vi "_AllThings.vi"   [LabVIEW 2017]
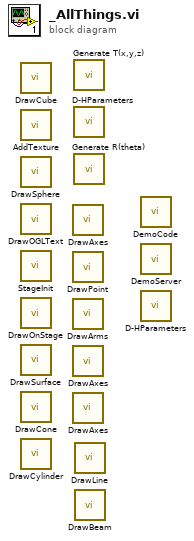
[diagram p0: block diagram]
diagram:
  n1 = call <userlib>:"DrawCube.vi"() -> ()  [unwired: 6 in, 2 out]
  n2 = call <userlib>:"AddTexture.vi"() -> ()  [unwired: 4 in, 2 out]
  n3 = call <userlib>:"DrawSphere.vi"() -> ()  [unwired: 6 in, 2 out]
  n4 = call <userlib>:"DrawOGLText.vi"() -> ()  [unwired: 6 in, 2 out]
  n5 = call <userlib>:"StageInit.vi"() -> ()  [unwired: 4 in, 2 out]
  n6 = call <userlib>:"DrawOnStage.vi"() -> ()  [unwired: 3 in, 3 out]
  n7 = call <userlib>:"DrawSurface.vi"() -> ()  [unwired: 6 in, 2 out]
  n8 = call <userlib>:"DrawCone.vi"() -> ()  [unwired: 6 in, 2 out]
  n9 = call <userlib>:"DrawCylinder.vi"() -> ()  [unwired: 6 in, 2 out]
  n10 = call <userlib>:"DrawAxes.vi"() -> ()  [unwired: 5 in, 1 out]
  n11 = call <userlib>:"DrawPoint.vi"() -> ()  [unwired: 3 in, 1 out]
  n12 = call <userlib>:"DrawArms.vi"() -> ()  [unwired: 6 in, 2 out]
  n13 = call <userlib>:"DrawAxes.vi"() -> ()  [unwired: 5 in, 1 out]
  n14 = call <userlib>:"DrawAxes.vi"() -> ()  [unwired: 5 in, 1 out]
  n15 = call <userlib>:"Generate T(x,y,z).vi"() -> ()  [unwired: 3 in, 1 out]
  n16 = call <userlib>:"D-HParameters.vi"() -> ()  [unwired: 3 in, 1 out]
  n17 = call <userlib>:"Generate R(theta).vi"() -> ()  [unwired: 3 in, 1 out]
  n18 = call <userlib>:"DrawLine.vi"() -> ()  [unwired: 5 in, 2 out]
  n19 = call <userlib>:"DrawBeam.vi"() -> ()  [unwired: 6 in, 1 out]
  n20 = call <userlib>:"DemoCode.vi"() -> ()  [unwired: 12 in]
  n21 = call <userlib>:"DemoServer.vi"() -> ()  [unwired: 12 in]
  n22 = call <userlib>:"D-HParameters.vi"() -> ()  [unwired: 3 in, 1 out]
